vi "FGGA Serial Data Server & Recordingv3.1_test.vi"() -> ()   [LabVIEW 2014]
uses:
  <vilib>/Instr/_visa.llb/VISA Set IO Buffer Mask.ctl
  <vilib>/Instr/_visa.llb/VISA Flush IO Buffer Mask.ctl
  <vilib>/Platform/TimedLoop/XDataNode/timing_clust.ctl
  <vilib>/Platform/TimedLoop/XDataNode/nitl_modes.ctl
  <vilib>/Platform/TimedLoop/XDataNode/wakeup.ctl
  C:/Program Files (x86)/National Instruments/LabVIEW 2014/examples/Data Communication/Network Streams/Simple Network Streams/support/Network Stream Command.ctl
  <vilib>/Utility/error.llb/whitespace.ctl
  <vilib>/Instr/_visa.llb/VISA Configure Serial Port (Instr).vi
  <vilib>/Utility/tcp.llb/UDP Multicast Write-Only Open.vi
  <vilib>/platform/TimedLoop/XDataNode/XDataNode.xnode
  <vilib>/Platform/TimedLoop/XDataNode/XDNodeRunTimeDep.lvlib
panel:
  out "date/time string":string
  out "FGGA Pump":bool
  out "Flight Number":string
  out "Stop File Write":bool
  out "Default file name":string
  out "MFC":dbl[](array[numeric])
  out "FGGA restart":bool
  out "V4":bool
  out "V3":bool
  out "V2":bool
  out "V1":bool
  out "error out 2":errorcluster
  out "error out":errorcluster
  in  "MFC_1 SLPM set value":dbl
  out "Value Read":string
  out "status":bool
  in  "VISA resource name":refnum<visa-resource-name>="ASRL3::INSTR"
  in  "timeout (10sec) 2":u32=3000
  out "Labview_Viewer_UDP_Error_Out":errorcluster
  in  "Clear Display\nErrors":bool
  out "Data Processing":bool
  out "TCP Binary Packet":string
  in  "Time Stamp\nOffset":u32=1
  out "Data String":string
  out "UDP_ACSII_Out":string
  out "Serial error out":errorcluster
  out "SEPTIC TCP Error Out":errorcluster
  out "TCP packet\nSend To SEPTIC":bool
  out "FISH TCP Error Out":errorcluster
  out "TCP packet\nSend To FISH":bool
  out "UDP_Pack_num":u32
  out "UDP_Out Status":bool
  out "UDP_Out_Error Out":errorcluster
  out "Data Array":string[](array[string])
  out "RAW DATA":string
  in  "stop":bool
  in  "timeout (10sec)":u32=1500
  in  "VISA resource name":refnum<visa-resource-name>="ASRL7::INSTR"
  out "Number of times \nRead time out":u32
  out "Loop count":i32
  # "Date"
  # "Time"
  # "CH4"
  # "CO2"
  # "H2O"
  # "Cell Pressure"
  # "Cell Temperature"
  # "Spectral Flag"
  # "Ring Down Time (Laser A)"
  # "Ring Down Time (Laser B)"
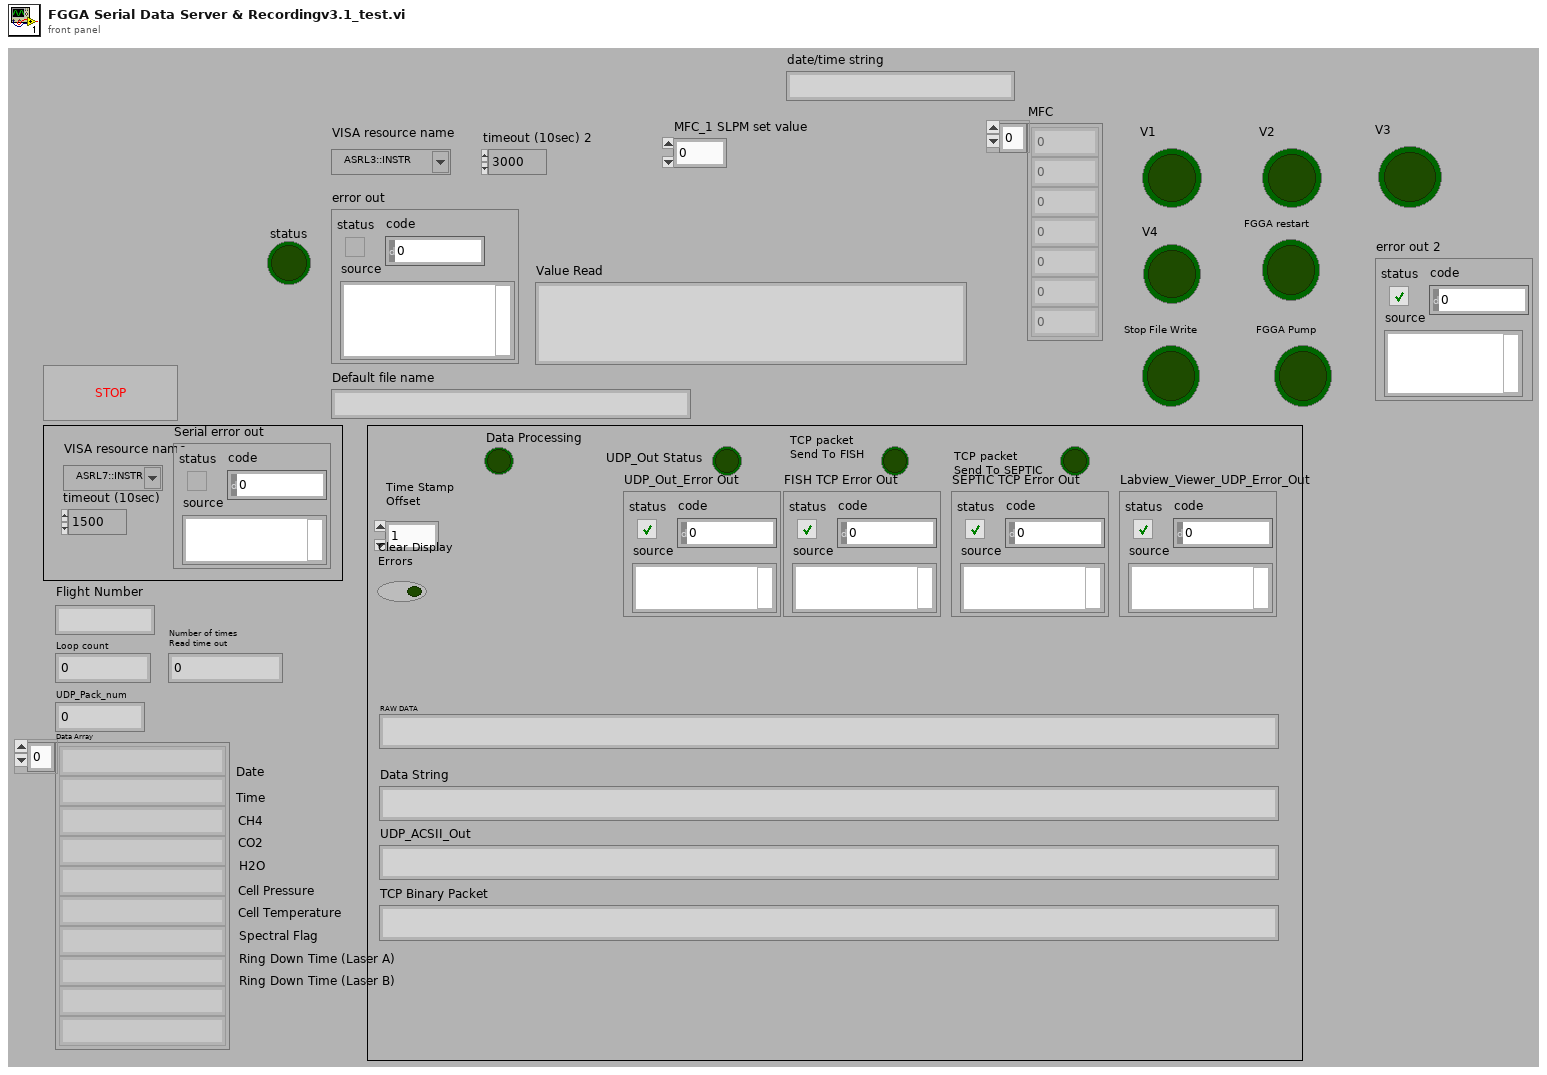
[diagram p1: front panel]
types:
  T1 = typedef "VISA Flush IO Buffer Mask.ctl" = u16
  T2 = typedef "VISA Set IO Buffer Mask.ctl" = u16
  T3 = typedef "XDNodeRunTimeDep.lvlib/timing_clust.ctl" = cluster{"Expected End [f-1]":u64, "Actual End [f-1]":u64, "Finished Late? [f-1]":bool, "Expected End [i-1]":u64, "Actual End [i-1]":u64, "Finished Late? [i-1]":bool, "Expected Start [i]":u64, "Actual Start [i]":u64, "Expected Start [f]":u64, "Actual Start [f]":u64, "Source Name":string, "Structure Name":string, "Period":i64, "Deadline":i64, "Offset":i64, "Start":i64, "Priority":i32, "Timeout":i32, "Mode":T4, "Wakeup Reason":T5, "Error":errorcluster, "Source Type":string, "Secondary Source Type":string, "Global End Time":u64, "Global Start Time":u64, "Frame Duration":u64, "Iteration Duration":u64, "Assigned CPU":i32, "I/O Scan Engine Mode":u32}
  T4 = typedef "XDNodeRunTimeDep.lvlib/nitl_modes.ctl" = enum32{"No Change", "Process missed periods, maintain original phase", "Discard missed periods, maintain original phase", "Process missed periods, ignore original phase", "Discard missed periods, ignore original phase"}
  T5 = typedef "XDNodeRunTimeDep.lvlib/wakeup.ctl" = enum32{"Normal", "Aborted", "Asynchronous wakeup", "Timing source error", "Timed loop error", "Timeout"}
  T6 = typedef "Network Stream Command.ctl" = cluster{"Message":string, "Message Data":variant}
  T7 = enum16{"open", "replace", "create", "open or create", "replace or create", "replace or create with confirmation"}
  T8 = typedef "whitespace.ctl" = u16
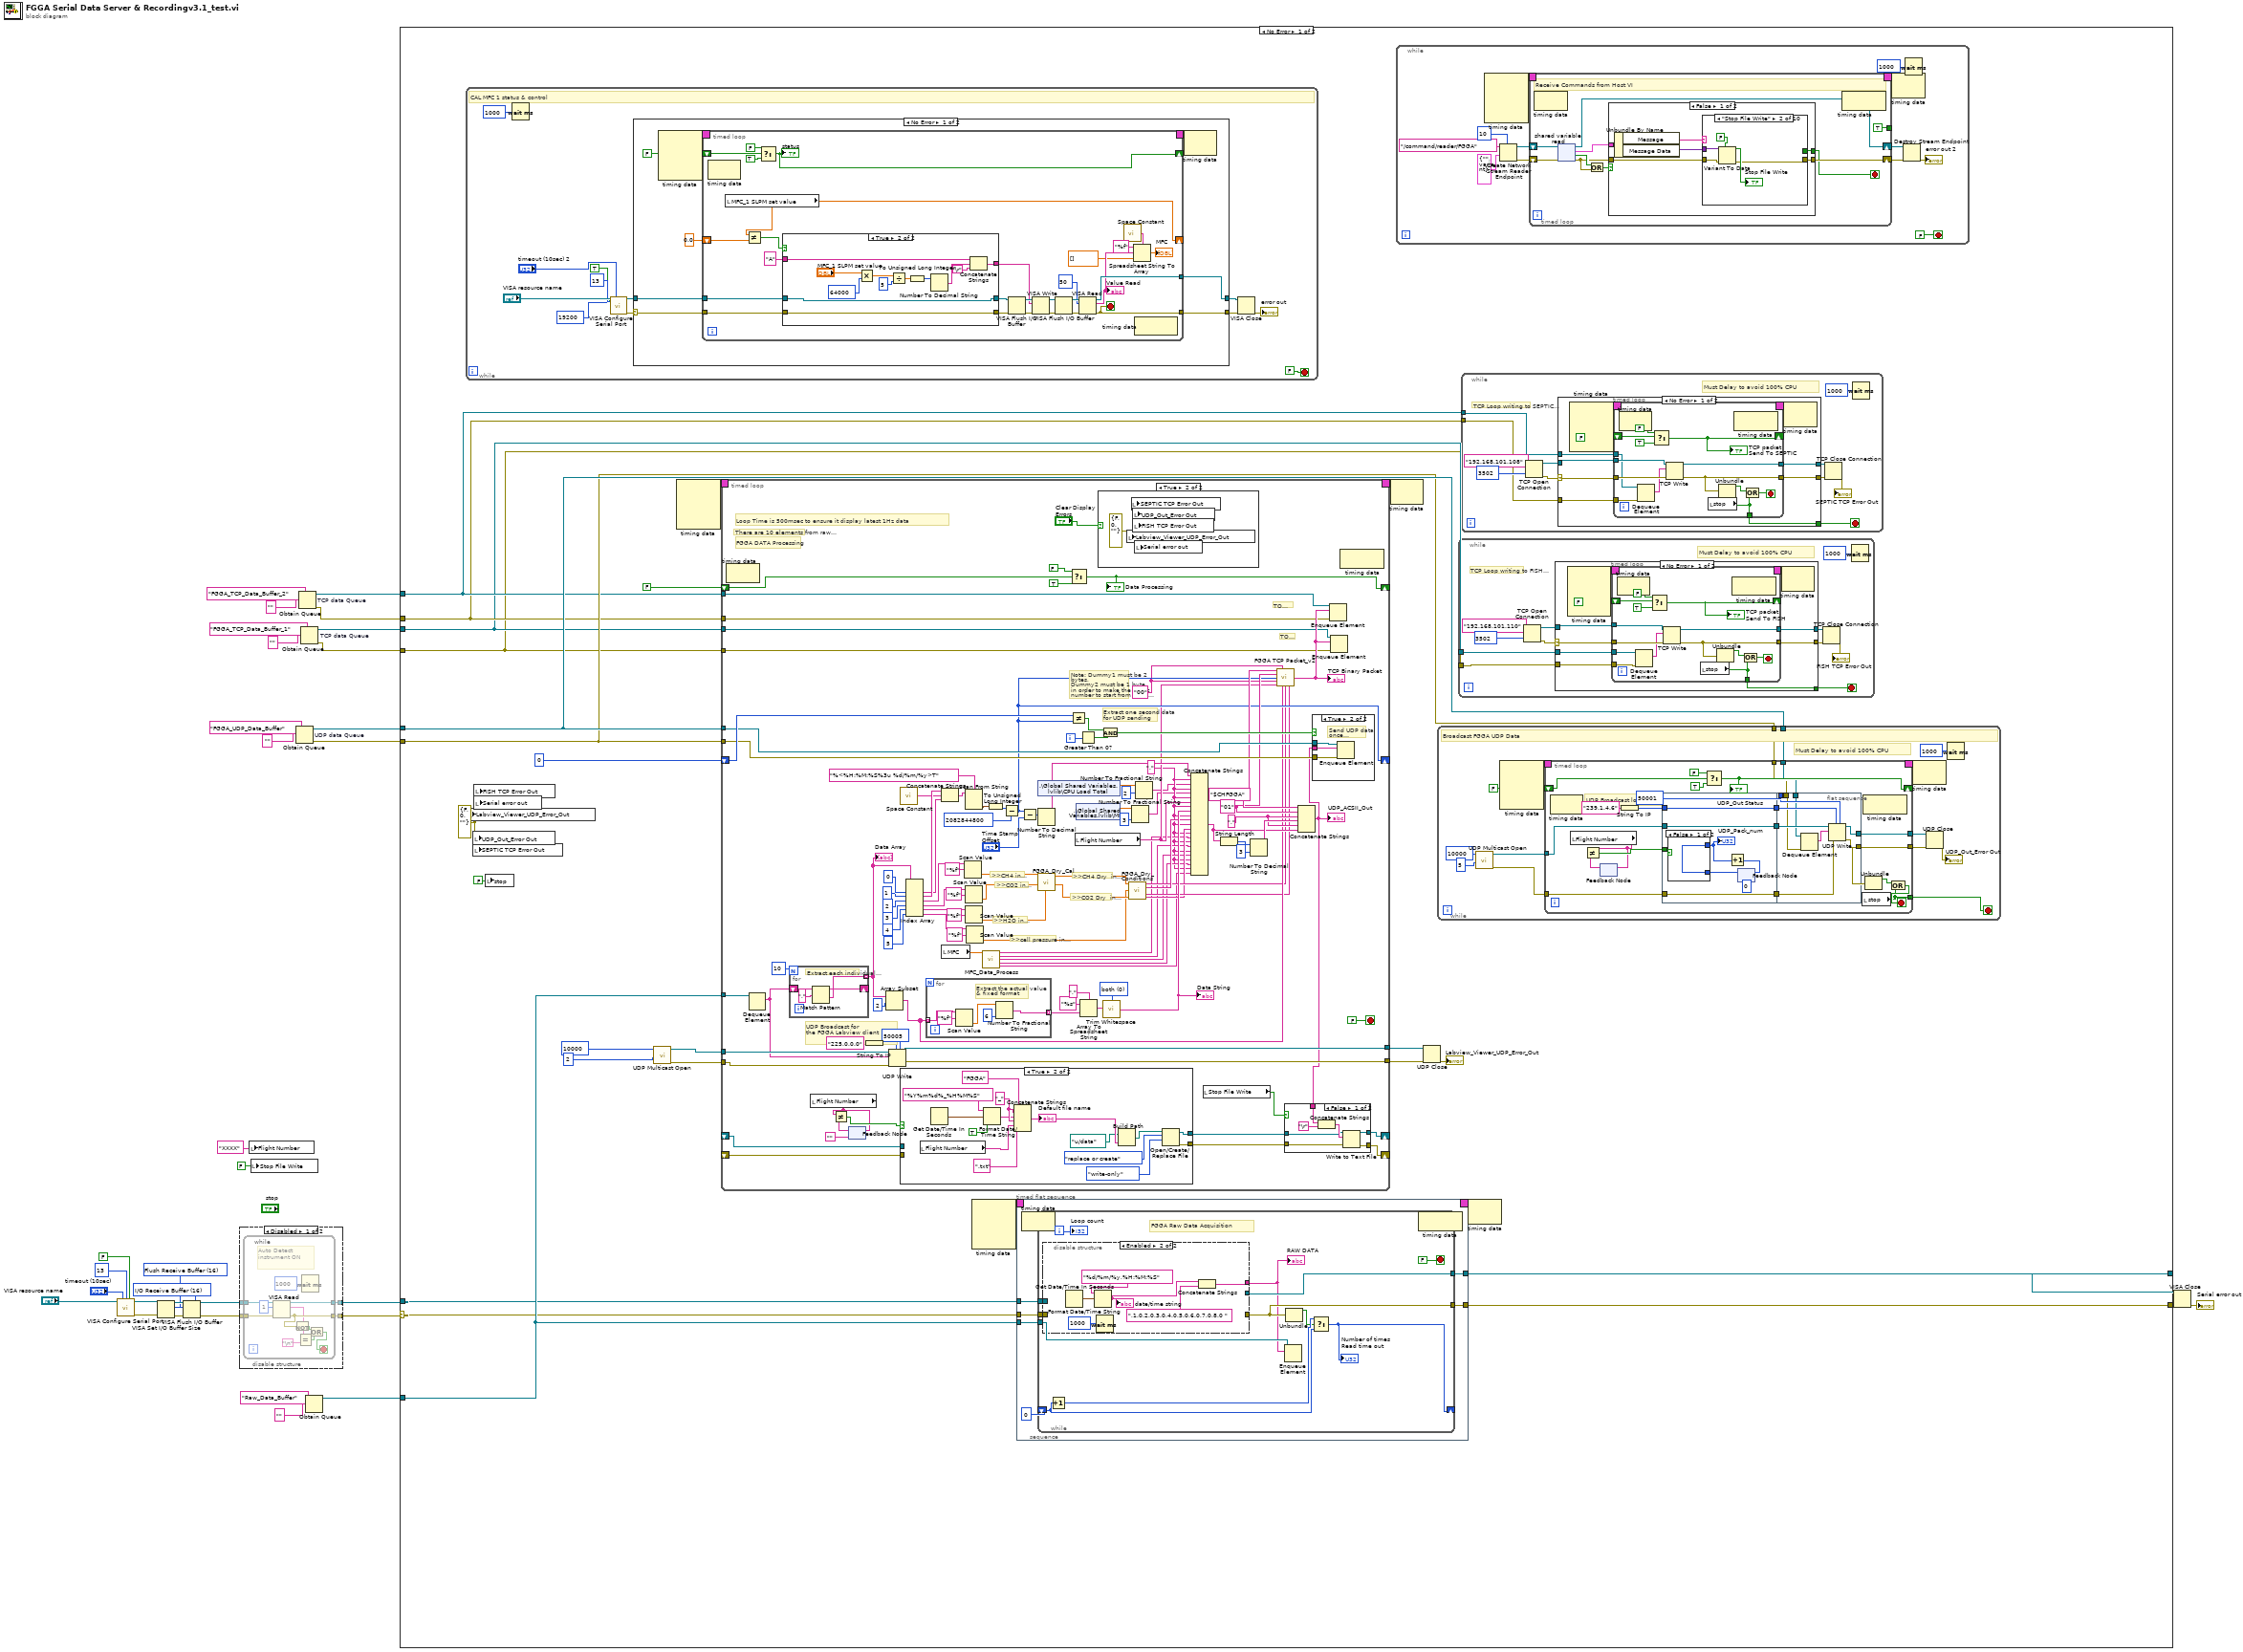
[diagram p0: block diagram]
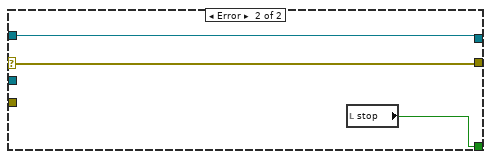
[diagram p3: hidden frame]
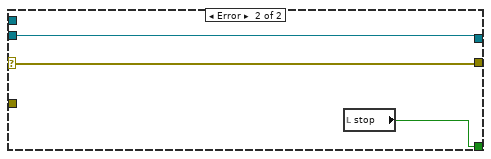
[diagram p4: hidden frame]
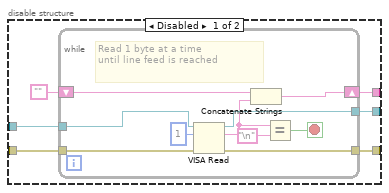
[diagram p5: hidden frame]
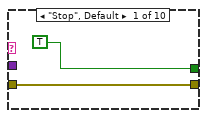
[diagram p6: hidden frame]
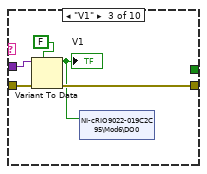
[diagram p7: hidden frame]
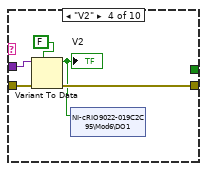
[diagram p8: hidden frame]
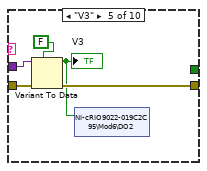
[diagram p9: hidden frame]
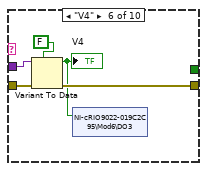
[diagram p10: hidden frame]
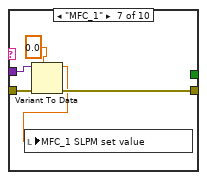
[diagram p11: hidden frame]
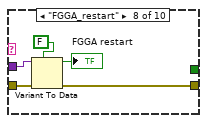
[diagram p12: hidden frame]
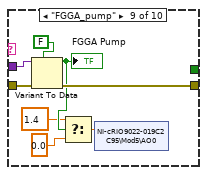
[diagram p13: hidden frame]
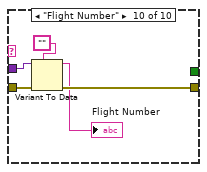
[diagram p14: hidden frame]
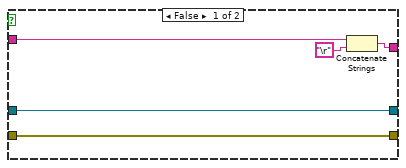
[diagram p16: hidden frame]
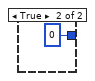
[diagram p18: hidden frame]
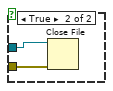
[diagram p20: hidden frame]
diagram:
  w9 = T1 16 items=["Flush Receive Buffer"=16, "Write Transmit Buffer to Device"=32, "Flush Receive Buffer (No I/O)"=64, "Flush Transmit Buffer"=128] ("Mask")
  w10 = T2 16 items=["I/O Receive Buffer"=16, "I/O Transmit Buffer"=32, "I/O Receive and Transmit Buffer"=48] ("Mask")
  n1 = call-poly "VISA Configure Serial Port"("VISA resource name"="VISA resource name", "timeout (10sec)"="timeout (10sec)", "termination char\n(0xA = '\\n' = LF)"=u8 13 ("termination char\n(0xA = '\\n' = LF)"), "Enable Termination\nChar (T)"=FALSE ("Enable Termination\nChar (T)")) -> ("VISA resource name out"=w8:refnum<visa-resource-name>, "error out"=w7:errorcluster)  [unwired: 10 in]
  n2 = VISA Set I/O Buffer Size(VISA resource name=w8, mask (16)=w10, error in (no error)=w7) -> (VISA resource name out=w11:refnum<visa-resource-name>, error out=w12:errorcluster)  [unwired: 1 in]
  n3 = VISA Flush I/O Buffer(VISA resource name=w11, mask (16)=w9, error in (no error)=w12) -> (VISA resource name out=w6:refnum<visa-resource-name>, error out=w5:errorcluster)
  n4 = disable-structure shown="Disabled" {
    disable-tunnel: w6 -> [w38 _]
    disable-tunnel: w5 -> [w37 _]
    disable-tunnel: [w36 _] -> w4
    disable-tunnel: [w35 _] -> w3
    frame Disabled {
      n5 = while {
        tunnel: w38 -> [w49]
        tunnel: w37 -> [w48]
        tunnel: [w46] -> w36
        tunnel: [w45] -> w35
        stop <- w40 stop-if-true
        # "Auto Detect\ninstrument ON"
        n6 = VISA Read(VISA resource name=w49, byte count=u32 1, error in (no error)=w48) -> (VISA resource name out=w45:refnum<visa-resource-name>, read buffer=w43:string, error out=w46:errorcluster)  [unwired: 1 out]
        n7 = Not(x=w46) -> (.not. x?=w42:bool)
        n8 = Equal?(x=w43, y="\n") -> (x = y?=w41:bool)
        n9 = Wait (ms)(milliseconds to wait=u32 1000) -> ()  [unwired: 1 out]
        n10 = Or(x=w42, y=w41) -> (x .or. y?=w40:bool)
      }
    }
    frame Enabled {
    }
  }
  n11 = local write "Flight Number"("XXXX" ("Flight Number")) -> ()
  n12 = local write "Stop File Write"(FALSE ("Stop File Write")) -> ()
  n13 = Obtain Queue "UDP data Queue"(name (unnamed)="FGGA_UDP_Data_Buffer", element data type="") -> (queue out=w22:refnum<queue>, error out=w21:errorcluster)  [unwired: 3 in, 1 out]
  n14 = Obtain Queue "TCP data Queue"(name (unnamed)="FGGA_TCP_Data_Buffer_2", element data type="") -> (queue out=w16:refnum<queue>, error out=w15:errorcluster)  [unwired: 3 in, 1 out]
  n15 = Obtain Queue "TCP data Queue"(name (unnamed)="FGGA_TCP_Data_Buffer_1", element data type="") -> (queue out=w14:refnum<queue>, error out=w13:errorcluster)  [unwired: 3 in, 1 out]
  n16 = Obtain Queue(name (unnamed)="Raw_Data_Buffer", element data type="") -> (queue out=w28:refnum<queue>)  [unwired: 3 in, 2 out]
  n17 = case shown="No Error" w4 {
    selector: w4 -> [w52 w572]
    tunnel: w3 -> [w53 w573]
    tunnel: [w74 w573] -> w25
    tunnel: [w75 w572] -> w26
    tunnel: w28 -> [w71 _]
    tunnel: w22 -> [w69 _]
    tunnel: w21 -> [w68 _]
    tunnel: w16 -> [w67 _]
    tunnel: w15 -> [w66 _]
    tunnel: w14 -> [w65 _]
    tunnel: w13 -> [w64 _]
    frame No Error {
      w55 = errorcluster {"status"=FALSE, "code"=0, "source"=""} ("UDP Error Out")
      n18 = while {
        stop <- FALSE stop-if-true
        # "CAL MFC 1 status & control"
        n19 = Wait (ms)(milliseconds to wait=u32 1000) -> ()  [unwired: 1 out]
        n20 = call-poly "VISA Configure Serial Port"("VISA resource name"="VISA resource name", "timeout (10sec)"="timeout (10sec) 2", "termination char\n(0xA = '\\n' = LF)"=u8 13 ("termination char\n(0xA = '\\n' = LF)"), "Enable Termination\nChar (T)"=TRUE ("Enable Termination\nChar (T)"), "baud rate (9600)"=u32 19200) -> ("VISA resource name out"=w304:refnum<visa-resource-name>, "error out"=w300:errorcluster)  [unwired: 9 in]
        n21 = case shown="No Error" w300 {
          selector: w300 -> [w311 w361]
          tunnel: w304 -> [w312 w362]
          tunnel: [w310 w362] -> w303
          tunnel: [w309 w361] -> w302
          frame No Error {
            n22 = node-c288() -> (w307:T3)  [unwired: 4 in]
            n23 = timed-loop {
              tunnel: w312 -> [w335]
              tunnel: w311 -> [w333]
              tunnel: [w326] -> w310
              tunnel: [w321] -> w309
              shift-right: [w322] -> _
              shift-left: FALSE -> [w325]
              timing: w307 -> [_]
              timing-out: [_] -> w306
              shift-right: [w313] -> _
              shift-left: 0.0 -> [w315]
              stop <- w321 stop-if-true
              n24 = node-c288() -> ()  [unwired: 1 in, 1 out]
              n25 = local read "MFC_1 SLPM set value"() -> (w313:dbl)
              n26 = Not Equal?(x=w313, y=w315) -> (x != y?=w314:bool)
              n27 = Select(t=FALSE, s=w325, f=TRUE) -> (s? t:f=w322:bool)
              "status" <- w322
              n28 = case shown="True" w314 {
                tunnel: w335 -> [w343 w358]
                tunnel: [w343 w358] -> w334
                tunnel: w333 -> [w342 w357]
                tunnel: [w342 w357] -> w332
                tunnel: "A" -> [w346 w350]
                tunnel: [w344 w347] -> w330
                frame False {
                  n29 = Concatenate Strings(w346, "\r") -> (w344:string)
                }
                frame True {
                  n30 = Multiply(x="MFC_1 SLPM set value", y=u32 64000) -> (x*y=w354:dbl)
                  n31 = Divide(x=w354, y=u32 5) -> (x/y=w352:dbl)
                  n32 = To Unsigned Long Integer(number=w352) -> (unsigned 32bit integer=w351:u32)
                  n33 = Number To Decimal String(number=w351) -> (decimal integer string=w349:string)  [unwired: 1 in]
                  n34 = Concatenate Strings(w350, w349, "\r") -> (w347:string)
                }
              }
              n35 = VISA Flush I/O Buffer(VISA resource name=w334, error in (no error)=w332) -> (VISA resource name out=w337:refnum<visa-resource-name>, error out=w336:errorcluster)  [unwired: 1 in]
              n36 = VISA Write(VISA resource name=w337, write buffer=w330, error in (no error)=w336) -> (VISA resource name out=w329:refnum<visa-resource-name>, error out=w328:errorcluster)  [unwired: 1 out]
              n37 = VISA Flush I/O Buffer(VISA resource name=w329, error in (no error)=w328) -> (VISA resource name out=w339:refnum<visa-resource-name>, error out=w338:errorcluster)  [unwired: 1 in]
              n38 = VISA Read(VISA resource name=w339, byte count=u32 50, error in (no error)=w338) -> (VISA resource name out=w326:refnum<visa-resource-name>, read buffer=w320:string, error out=w321:errorcluster)  [unwired: 1 out]
              "Value Read" <- w320
              n39 = call <vilib>:"Space Constant.vi"() -> ("String"=w319:string)
              n40 = Spreadsheet String To Array(delimiter (Tab)=w319, format string="%f", spreadsheet string=w320, array type (2D Dbl)=dbl[] []) -> (array=→"MFC":dbl[])
              n41 = node-c288() -> ()  [unwired: 1 in, 1 out]
            }
            n42 = node-c288(w306) -> ()  [unwired: 1 out]
          }
          frame Error {
          }
        }
        n43 = VISA Close(VISA resource name=w303, error in (no error)=w302) -> (error out=→"error out":errorcluster)
      }
      n44 = local write "Labview_Viewer_UDP_Error_Out"(w55) -> ()
      n45 = local write "UDP_Out_Error Out"(w55) -> ()
      n46 = local write "SEPTIC TCP Error Out"(w55) -> ()
      n47 = local write "FISH TCP Error Out"(w55) -> ()
      n48 = local write "Serial error out"(w55) -> ()
      n49 = local write "stop"(FALSE ("stop")) -> ()
      n50 = call-poly <vilib>:"UDP Multicast Open.vi"("time-to-live (1)"=u16 2, "port"=u16 10000) -> ("error out"=w59:errorcluster, "connection ID"=w60:refnum<k16>)  [unwired: 8 in]
      n51 = node-c288() -> (w73:T3)  [unwired: 4 in]
      n52 = timed-loop {
        timing: w73 -> [_]
        timing-out: [_] -> w72
        tunnel: w71 -> [w528]
        tunnel: w69 -> [w483]
        tunnel: w68 -> [w482]
        shift-right: [w479] -> _
        shift-left: u32 0 -> [w486]
        tunnel: w67 -> [w474]
        tunnel: w66 -> [w473]
        tunnel: w65 -> [w472]
        tunnel: w64 -> [w471]
        shift-right: [w467] -> _
        shift-left: FALSE -> [w470]
        tunnel: w60 -> [w463]
        tunnel: w59 -> [w462]
        tunnel: [w461] -> w58
        tunnel: [w460] -> w57
        shift-right: [w439] -> _
        shift-left: _ -> [w431]
        shift-right: [w429] -> _
        shift-left: _ -> [w430]
        i -> [w485]
        stop <- FALSE stop-if-true
        w478 = "00"
        w441 = ","
        w514 = T8 0 items=["both", "start of string", "end of string"] ("location (both)")
        w522 = ","
        w480 = "01"
        w481 = "$CHFGGA"
        # "Note: Dummy1 must be 2 bytes, \nDummy2 must be 1 byte\nin order to make the Flight \nnumber to start from byte 20\n(this only applies to TCP packet)"
        # ">>cell pressure in torr>>"
        # "UDP Broadcast for\nthe FGGA Labview client"
        # "There are 10 elements from raw packet"
        # "TO SEPTIC"
        # "TO FISH"
        # "Extract one second data\nfor UDP sending"
        # ">>CO2 Dry  in ppm>>"
        # ">>CH4 Dry  in ppb>>"
        # ">>H2O in ppm>>"
        # ">>CO2 in ppm>>"
        # ">>CH4 in ppm>>"
        # "Loop Time is 500msec to ensure it display latest 1Hz data"
        # "FGGA DATA Processing"
        n53 = node-c288() -> ()  [unwired: 1 in, 1 out]
        n54 = Dequeue Element(queue=w528) -> (element=w459:string)  [unwired: 2 in, 3 out]
        n55 = for {
          N: 10 -> [_]
          shift-right: [w566] -> _
          shift-left: w459 -> [w564]
          tunnel: [w565] -> w519 mode=indexing
          # "Extract each individual param"
          n56 = Match Pattern(string=w564, regular expression=",") -> (before substring=w565:string, after substring=w566:string)  [unwired: 1 in, 2 out]
        }
        "Data Array" <- w519
        n57 = local read "Flight Number"() -> (w428:string)
        n58 = feedback #1("" ("Flight Number")) -> (w436:string)
        n59 = Not Equal?(x=w428, y=w436) -> (x != y?=w434:bool)
        n60 = feedback-in #1(w428) -> ()
        n61 = String To IP(1:"225.0.0.0" ("name")) -> (0:w464:u32)
        n62 = Array Subset(array=w519, index=2) -> (w476:string[])  [unwired: 1 in]
        n63 = UDP Write(address=w464, port or service name=u16 50005, connection ID=w463, data in=w459, 8:w462) -> (error out=w460:errorcluster, 3:w461:refnum<k16>)  [unwired: 1 in]
        n64 = case shown="True" w434 {
          tunnel: [w530 w532] -> w433
          tunnel: [w529 w531] -> w432
          tunnel: w431 -> [w530 _]
          tunnel: w430 -> [w529 _]
          frame False {
          }
          frame True {
            w538 = "_" ("string")
            n65 = local read "Flight Number"() -> (w545:string)
            n66 = Get Date/Time In Seconds() -> (seconds since 1Jan1904=w533:timestamp)
            n67 = Format Date/Time String(time format string (%c)="%Y%m%d%_%H%M%S", seconds (now)=w533, UTC format=TRUE) -> (date/time string=w535:string)
            n68 = Concatenate Strings("FGGA" ("string"), w538, w535, w538, w545, ".txt" ("string")) -> (w540:string)
            "Default file name" <- w540
            n69 = Build Path(base path=path "u:/data", name or relative path=w540) -> (appended path=w544:path)
            n70 = Open/Create/Replace File(file path (use dialog)=w544, operation (0:open)=T7."replace or create", access (0:read/write)=enum16{"read/write", "read-only", "write-only"}."write-only") -> (refnum out=w532:refnum<file>, error out=w531:errorcluster)  [unwired: 3 in, 1 out]
          }
        }
        n71 = call <vilib>:"Space Constant.vi"() -> ("String"=w497:string)
        n72 = Index Array(array=w519, index #1=0 ("index"), index #2=1 ("index"), index #3=2 ("index"), index #4=3 ("index"), index #5=4 ("index"), index #6=5 ("index")) -> (element #1=w496:string, element #2=w498:string, element #3=w502:string, element #4=w501:string, element #5=w500:string, element #6=w450:string)
        n73 = for {
          tunnel: w476 -> [w562] mode=indexing
          tunnel: [w559] -> w512 mode=indexing
          # "Extract the actual value\n& fixed format"
          n74 = Scan Value(string=w562, format string="%f") -> (value=w560:dbl)  [unwired: 1 in, 1 out]
          n75 = Number To Fractional String(number=w560, precision (6)=i16 6) -> (F-format string=w559:string)  [unwired: 2 in]
        }
        n76 = Concatenate Strings(w498, w497, w496) -> (w495:string)
        n77 = local read "MFC"() -> (w446:dbl[])
        n78 = Scan Value(string=w502, format string="%f") -> (value=w504:dbl)  [unwired: 1 in, 1 out]
        n79 = Scan Value(string=w501, format string="%f") -> (value=w503:dbl)  [unwired: 1 in, 1 out]
        n80 = Scan From String(format string="%<%H:%M:%S%3u %d/%m/%y>T", input string=w495) -> (output 1=w492:timestamp)  [unwired: 3 in, 3 out]
        n81 = Scan Value(string=w500, format string="%f") -> (value=w447:dbl)  [unwired: 1 in, 1 out]
        n82 = Scan Value(string=w450, format string="%f") -> (value=w448:dbl)  [unwired: 1 in, 1 out]
        n83 = call "MFC_Data_Process.vi"("MFC"=w446) -> ("MFC Absolute Pressure"=w445:string, "MFC Temperature"=w444:string, "MFC Volumetric Flow"=w443:string, "MFC Mass Flow"=w442:string, "MFC Set Point"=w440:string)  [unwired: 10 in]
        n84 = To Unsigned Long Integer(number=w492) -> (unsigned 32bit integer=w493:u32)
        n85 = Subtract(x=w493, y=u32 2082844800) -> (x-y=w479:u32)
        n86 = Subtract(x=w479, y="Time Stamp\nOffset") -> (x-y=w489:u32)
        n87 = shared-variable ".\\Global Shared Variables.lvlib\\CPU Load Total"() -> (w427:dbl)  [unwired: 1 in, 1 out]
        n88 = Number To Decimal String(number=w489) -> (decimal integer string=w491:string)  [unwired: 1 in]
        n89 = call "FGGA_Dry_Cal.vi"("H2O"=w447, "CO2_Wet"=w503, "CH4_Wet"=w504) -> ("CO2_Dry"=w452:dbl, "CH4_Dry"=w454:dbl)  [unwired: 7 in]
        n90 = Select(t=FALSE, s=w470, f=TRUE) -> (s? t:f=w467:bool)
        "Data Processing" <- w467
        n91 = Not Equal?(x=w486, y=w479) -> (x != y?=w487:bool)
        n92 = local read "Flight Number"() -> (w477:string)
        n93 = shared-variable ".\\Global Shared Variables.lvlib\\MFM"() -> (w424:dbl)  [unwired: 1 in, 1 out]
        n94 = Greater Than 0?(x=w485) -> (x > 0?=w488:bool)
        n95 = Array To Spreadsheet String(delimiter (Tab)=",", array=w512, 3:"%s" ("format string")) -> (spreadsheet string=w513:string)
        n96 = case shown="True" "Clear Display\nErrors" {
          frame False {
          }
          frame True {
            w555 = errorcluster {"status"=FALSE, "code"=0, "source"=""} ("UDP Error Out")
            n97 = local write "Labview_Viewer_UDP_Error_Out"(w555) -> ()
            n98 = local write "SEPTIC TCP Error Out"(w555) -> ()
            n99 = local write "UDP_Out_Error Out"(w555) -> ()
            n100 = local write "FISH TCP Error Out"(w555) -> ()
            n101 = local write "Serial error out"(w555) -> ()
          }
        }
        n102 = call <vilib>:"Trim Whitespace.vi"("string"=w513, "location (both)"=w514) -> ("trimmed string"=w511:string)
        "Data String" <- w511
        n103 = Compound Arithmetic op=AND(w487, w488) -> (w484:bool)
        n104 = call "FGGA_Dry_Conditions.vi"("CH4_Dry"=w454, "Pressure"=w448, "CO2_Dry"=w452) -> ("CH4_Dry_TCP"=w457:string, "CH4_Dry_UDP"=w458:string, "CO2_Dry_TCP"=w456:string, "CO2_Dry_UDP"=w455:string)  [unwired: 9 in]
        n105 = Number To Fractional String(number=w424, precision (6)=i16 3) -> (F-format string=w422:string)  [unwired: 2 in]
        n106 = Number To Fractional String(number=w427, precision (6)=i16 2) -> (F-format string=w425:string)  [unwired: 2 in]
        n107 = Concatenate Strings(w491, w441, w425, w441, w422, w441, w477, w441, w511, w441, w458, w441, w455, w441, w445, w441, w444, w441, w443, w441, w442, w441, w440) -> (w521:string)
        n108 = local read "Stop File Write"() -> (w437:bool)
        n109 = String Length(string=w521) -> (length=w525:i32)
        n110 = Number To Decimal String(number=w525, width (-)=i16 3) -> (decimal integer string=w523:string)
        n111 = call "FGGA TCP Packet_v2.vi"("ID"=w481, "dummy2"=w478, "Version"=w480, "utc_time"=w479, "dummy1"=w478, "Flight Number"=w477, "Data Array"=w476, "ch4_dry"=w457, "co2_dry"=w456) -> ("TCP Binary Packet"=w475:string)  [unwired: 6 in]
        "TCP Binary Packet" <- w475
        n112 = Concatenate Strings(w481, w480, w522, w523, w522, w521) -> (w438:string)
        "UDP_ACSII_Out" <- w438
        n113 = case shown="False" w437 {
          tunnel: w438 -> [w552 _]
          tunnel: [w549 _] -> w439
          tunnel: w433 -> [w548 w554]
          tunnel: w432 -> [w547 w553]
          tunnel: [w546 _] -> w429
          frame False {
            n114 = Concatenate Strings(w552, "\r") -> (w550:string)
            n115 = Write to Text File(file (use dialog)=w548, text=w550, error in=w547) -> (refnum out=w549:refnum<file>, error out=w546:errorcluster)  [unwired: 2 out]
          }
          frame True {
            n116 = Close File(refnum=w554, error in=w553) -> ()  [unwired: 2 out]
          }
        }
        n117 = case shown="True" w484 {
          tunnel: w438 -> [_ w558]
          tunnel: w483 -> [_ w557]
          tunnel: w482 -> [_ w556]
          frame False {
          }
          frame True {
            # "Send UDP data once\na second"
            n118 = Enqueue Element(queue=w557, element=w558, error in (no error)=w556) -> ()  [unwired: 1 in, 3 out]
          }
        }
        n119 = Enqueue Element(queue=w474, element=w475, error in (no error)=w473) -> ()  [unwired: 1 in, 3 out]
        n120 = Enqueue Element(queue=w472, element=w475, error in (no error)=w471) -> ()  [unwired: 1 in, 3 out]
        n121 = node-c288() -> ()  [unwired: 1 in, 1 out]
      }
      n122 = node-c288() -> (w51:T3)  [unwired: 4 in]
      n123 = timed-sequence {
        timing: w51 -> [_]
        timing-out: [_] -> w50
        tunnel: [w164] -> w75
        tunnel: [w163] -> w74
        tunnel: w71 -> [w162]
        tunnel: w53 -> [w161]
        tunnel: w52 -> [w160]
        n124 = timed-flat-sequence {
          tunnel: [w170] -> w164
          tunnel: [w169] -> w163
          tunnel: w162 -> [w167]
          tunnel: w161 -> [w166]
          tunnel: w160 -> [w165]
          n125 = node-c288() -> ()  [unwired: 1 in, 1 out]
          n126 = while {
            tunnel: w166 -> [w182]
            tunnel: w165 -> [w181]
            tunnel: [w180] -> w170
            shift-right: [w176] -> _
            shift-left: u32 0 -> [w177]
            tunnel: [w179] -> w169
            tunnel: w167 -> [w174]
            i -> [w178]
            stop <- FALSE stop-if-true
            # "FGGA Raw Data Acquisition"
            n127 = disable-structure shown="Enabled" {
              disable-tunnel: w182 -> [w188 _]
              disable-tunnel: w181 -> [w187 _]
              disable-tunnel: [w186 _] -> w180
              disable-tunnel: [w185 _] -> w179
              disable-tunnel: [w183 w200] -> w173
              frame Disabled {
                n128 = while {
                  tunnel: [w198] -> w185
                  tunnel: [w197] -> w186
                  tunnel: w188 -> [w196]
                  tunnel: w187 -> [w195]
                  shift-right: [w193] -> w183
                  shift-left: "" -> [w194]
                  stop <- w190 stop-if-true
                  # "Read 1 byte at a time \nuntil line feed is reached"
                  n129 = VISA Read(VISA resource name=w196, byte count=u32 1, error in (no error)=w195) -> (VISA resource name out=w198:refnum<visa-resource-name>, read buffer=w192:string, error out=w197:errorcluster)  [unwired: 1 out]
                  n130 = Concatenate Strings(w194, w192) -> (w193:string)
                  n131 = Equal?(x=w192, y="\n") -> (x = y?=w190:bool)
                }
              }
              frame Enabled {
                n132 = Get Date/Time In Seconds() -> (seconds since 1Jan1904=w203:timestamp)
                n133 = Format Date/Time String(time format string (%c)="%d/%m/%y,%H:%M:%S" ("format string"), seconds (now)=w203) -> (date/time string=w199:string)  [unwired: 1 in]
                "date/time string" <- w199
                n134 = Wait (ms)(milliseconds to wait=u32 1000) -> ()  [unwired: 1 out]
                n135 = Concatenate Strings(w199, ",1.0,2.0,3.0,4.0,5.0,6.0,7.0,8.0 " ("RAW DATA")) -> (w200:string)
              }
            }
            "RAW DATA" <- w173
            n136 = Increment(x=w177) -> (x+1=w175:u32)
            n137 = Enqueue Element(queue=w174, element=w173) -> ()  [unwired: 2 in, 3 out]
            n138 = Unbundle(w180) -> ("status"=w172:bool)  [unwired: 2 out]
            n139 = Select(t=w175, s=w172, f=w177) -> (s? t:f=w176:u32)
            "Number of times \nRead time out" <- w176
            "Loop count" <- w178
          }
          n140 = node-c288() -> ()  [unwired: 1 in, 1 out]
        }
      }
      n141 = node-c288(w72) -> ()  [unwired: 1 out]
      n142 = while {
        stop <- FALSE stop-if-true
        n143 = node-c288() -> (w210:T3)  [unwired: 4 in]
        n144 = Create Network Stream Reader Endpoint(7:10 ("reader buffer size"), 9:T6 {"Message"="", "Message Data"=variant} ("Message Cluster"), 11:"/command/reader/FGGA" ("reader url")) -> (0:w216:errorcluster, 3:w217:refnum<k21>)  [unwired: 4 in]
        n145 = timed-loop "Host->Target Command Reader" {
          shift-right: [w227] -> w214
          shift-left: w216 -> [w230]
          shift-right: [w228] -> w213
          shift-left: w217 -> [w229]
          tunnel: [TRUE] -> _
          timing: w210 -> [_]
          timing-out: [_] -> w209
          stop <- w221 stop-if-true
          # "Receive Commands from Host VI"
          n146 = node-c288() -> ()  [unwired: 1 in, 1 out]
          n147 = shared-variable-read(w229, w230) -> (w228:refnum<k21>, w223:errorcluster, w225:bool, w226:T6)  [unwired: 1 in]
          n148 = Or(x=w225, y=w223) -> (x .or. y?=w224:bool)
          n149 = case shown="False" w224 {
            selector: w224 -> [_ w289]
            tunnel: w223 -> [w238 w290]
            tunnel: [w237 w290] -> w227
            tunnel: w226 -> [w235 _]
            tunnel: [w236 w289] -> w221
            frame False {
              n150 = Unbundle By Name(w235) -> ("Message"=w234:string, "Message Data"=w233:variant)
              n151 = case shown="\"Stop File Write\"" w234 {
                tunnel: w238 -> [w240 w245 w250 w255 w260 w265 w270 w275 w283 w288]
                tunnel: [w240 w241 w249 w254 w259 w264 w269 w274 w282 w287] -> w237
                tunnel: w233 -> [_ w244 w248 w253 w258 w263 w268 w273 w281 w286]
                tunnel: [TRUE _ _ _ _ _ _ _ _ _] -> w236
                frame "Stop", Default {
                }
                frame "Stop File Write" {
                  n152 = Variant To Data(error in=w245, type=FALSE, Variant=w244) -> (data=→"Stop File Write":bool, error out=w241:errorcluster)
                }
                frame "V1" {
                  n153 = Variant To Data(error in=w250, type=FALSE, Variant=w248) -> (data=w246:bool, error out=w249:errorcluster)
                  "V1" <- w246
                  n154 = shared-variable "NI-cRIO9022-019C2C95\\Mod6\\DO0"(w246) -> ()  [unwired: 1 in, 1 out]
                }
                frame "V2" {
                  n155 = Variant To Data(error in=w255, type=FALSE, Variant=w253) -> (data=w251:bool, error out=w254:errorcluster)
                  "V2" <- w251
                  n156 = shared-variable "NI-cRIO9022-019C2C95\\Mod6\\DO1"(w251) -> ()  [unwired: 1 in, 1 out]
                }
                frame "V3" {
                  n157 = Variant To Data(error in=w260, type=FALSE, Variant=w258) -> (data=w256:bool, error out=w259:errorcluster)
                  "V3" <- w256
                  n158 = shared-variable "NI-cRIO9022-019C2C95\\Mod6\\DO2"(w256) -> ()  [unwired: 1 in, 1 out]
                }
                frame "V4" {
                  n159 = Variant To Data(error in=w265, type=FALSE, Variant=w263) -> (data=w261:bool, error out=w264:errorcluster)
                  "V4" <- w261
                  n160 = shared-variable "NI-cRIO9022-019C2C95\\Mod6\\DO3"(w261) -> ()  [unwired: 1 in, 1 out]
                }
                frame "MFC_1" {
                  n161 = Variant To Data(error in=w270, type=0.0, Variant=w268) -> (data=w266:dbl, error out=w269:errorcluster)
                  n162 = local write "MFC_1 SLPM set value"(w266) -> ()
                }
                frame "FGGA_restart" {
                  n163 = Variant To Data(error in=w275, type=FALSE, Variant=w273) -> (data=→"FGGA restart":bool, error out=w274:errorcluster)
                }
                frame "FGGA_pump" {
                  n164 = Variant To Data(error in=w283, type=FALSE, Variant=w281) -> (data=w278:bool, error out=w282:errorcluster)
                  "FGGA Pump" <- w278
                  n165 = Select(t=1.4 ("f"), s=w278, f=0.0 ("t")) -> (s? t:f=w279:dbl)
                  n166 = shared-variable "NI-cRIO9022-019C2C95\\Mod5\\AO0"(w279) -> ()  [unwired: 1 in, 1 out]
                }
                frame "Flight Number" {
                  n167 = Variant To Data(error in=w288, type="", Variant=w286) -> (data=→"Flight Number":string, error out=w287:errorcluster)
                }
              }
            }
            frame True {
            }
          }
          n168 = node-c288() -> ()  [unwired: 1 in, 1 out]
        }
        n169 = node-c288(w209) -> ()  [unwired: 1 out]
        n170 = Destroy Stream Endpoint(8:w214, 11:w213) -> (0:→"error out 2":errorcluster)
        n171 = Wait (ms)(milliseconds to wait=u32 1000) -> ()  [unwired: 1 out]
      }
      n172 = UDP Close(connection ID=w58, 8:w57) -> (error out=→"Labview_Viewer_UDP_Error_Out":errorcluster)  [unwired: 1 out]
      n173 = while {
        tunnel: w69 -> [w365]
        tunnel: w68 -> [w364]
        stop <- w366 stop-if-true
        # "Must Delay to avoid 100% CPU"
        # "Broadcast FGGA UDP Data"
        n174 = call-poly <vilib>:"UDP Multicast Open.vi"("time-to-live (1)"=u16 5, "port"=u16 10000) -> ("error out"=w373:errorcluster, "connection ID"=w374:refnum<k16>)  [unwired: 8 in]
        n175 = node-c288() -> (w376:T3)  [unwired: 4 in]
        n176 = timed-loop {
          tunnel: w374 -> [w397]
          tunnel: w373 -> [w396]
          timing: w376 -> [_]
          timing-out: [_] -> w375
          shift-right: [w385] -> _
          shift-left: FALSE -> [w388]
          tunnel: [w384] -> w368
          tunnel: [w382] -> w367
          tunnel: [w380] -> w366
          tunnel: w365 -> [w378]
          tunnel: w364 -> [w377]
          stop <- w381 stop-if-true
          # "UDP Broadcast loop"
          n177 = node-c288() -> ()  [unwired: 1 in, 1 out]
          n178 = local read "Flight Number"() -> (w379:string)
          n179 = feedback-in #2(w379) -> ()
          n180 = feedback #2() -> (w390:string)  [unwired: 1 in]
          n181 = Not Equal?(x=w379, y=w390) -> (x != y?=w389:bool)
          n182 = String To IP(1:"239.1.4.6" ("name")) -> (0:w394:u32)
          n183 = flat-sequence {
            tunnel: w394 -> [w404]
            tunnel: w396 -> [w405]
            tunnel: w397 -> [w406]
            tunnel: [w406] -> w393
            tunnel: [w405] -> w392
            tunnel: [w404] -> w391
            tunnel: w389 -> [w403]
            tunnel: u16 50001 ("port or service name") -> [w417]
            tunnel: w393 -> [w416]
            tunnel: w392 -> [w415]
            tunnel: w391 -> [w414]
            tunnel: [w413] -> w384
            tunnel: [w412] -> w382
            tunnel: w378 -> [w410]
            tunnel: w377 -> [w409]
            frame #0 {
              n184 = feedback #3(u32 0) -> (w400:u32)
              n185 = case shown="False" w403 {
                tunnel: w400 -> [w407 _]
                tunnel: [w407 u32 0] -> w399
                frame False {
                }
                frame True {
                }
              }
              "UDP_Pack_num" <- w399
              n186 = Increment(x=w399) -> (x+1=w401:u32)
              n187 = feedback-in #3(w401) -> ()
            }
            frame #1 {
              n188 = Dequeue Element(queue=w410, error in (no error)=w409) -> (element=w411:string)  [unwired: 1 in, 3 out]
              n189 = UDP Write(address=w414, port or service name=w417, connection ID=w416, data in=w411, 8:w415) -> (error out=w412:errorcluster, 3:w413:refnum<k16>)  [unwired: 1 in]
            }
          }
          n190 = Select(t=FALSE, s=w388, f=TRUE) -> (s? t:f=w385:bool)
          "UDP_Out Status" <- w385
          n191 = local read "stop"() -> (w380:bool)
          n192 = node-c288() -> ()  [unwired: 1 in, 1 out]
          n193 = Unbundle(w382) -> ("status"=w383:bool)  [unwired: 2 out]
          n194 = Compound Arithmetic op=OR(w383, w380) -> (w381:bool)
        }
        n195 = node-c288(w375) -> ()  [unwired: 1 out]
        n196 = UDP Close(connection ID=w368, 8:w367) -> (error out=→"UDP_Out_Error Out":errorcluster)  [unwired: 1 out]
        n197 = Wait (ms)(milliseconds to wait=u32 1000) -> ()  [unwired: 1 out]
      }
      n198 = while {
        tunnel: w65 -> [w78]
        tunnel: w64 -> [w77]
        stop <- w81 stop-if-true
        # "Must Delay to avoid 100% CPU"
        # "TCP Loop writing to FISH Tank"
        n199 = TCP Open Connection(address="192.168.101.110", remote port or service name=u16 3502) -> (connection ID=w84:refnum<k5>, error out=w79:errorcluster)  [unwired: 3 in]
        n200 = case shown="No Error" w79 {
          selector: w79 -> [w89 w116]
          tunnel: w84 -> [w94 w117]
          tunnel: [w93 w117] -> w83
          tunnel: [w92 w116] -> w82
          tunnel: [w91 w115] -> w81
          tunnel: w78 -> [w88 _]
          tunnel: w77 -> [w87 _]
          frame No Error {
            n201 = node-c288() -> (w96:T3)  [unwired: 4 in]
            n202 = timed-loop {
              tunnel: w94 -> [w110]
              tunnel: w89 -> [w109]
              tunnel: [w108] -> w93
              tunnel: [w107] -> w92
              tunnel: [w99] -> w91
              shift-right: [w101] -> _
              shift-left: FALSE -> [w104]
              timing: w96 -> [_]
              timing-out: [_] -> w95
              tunnel: w88 -> [w98]
              tunnel: w87 -> [w97]
              stop <- w105 stop-if-true
              n203 = node-c288() -> ()  [unwired: 1 in, 1 out]
              n204 = Dequeue Element(queue=w98, error in (no error)=w97) -> (element=w100:string)  [unwired: 1 in, 3 out]
              n205 = Select(t=FALSE, s=w104, f=TRUE) -> (s? t:f=w101:bool)
              "TCP packet\nSend To FISH" <- w101
              n206 = TCP Write(connection ID=w110, data in=w100, error in (no error)=w109) -> (connection ID out=w108:refnum<k5>, error out=w107:errorcluster)  [unwired: 1 in, 1 out]
              n207 = local read "stop"() -> (w99:bool)
              n208 = Unbundle(w107) -> ("status"=w106:bool)  [unwired: 2 out]
              n209 = node-c288() -> ()  [unwired: 1 in, 1 out]
              n210 = Compound Arithmetic op=OR(w106, w99) -> (w105:bool)
            }
            n211 = node-c288(w95) -> ()  [unwired: 1 out]
          }
          frame Error {
            n212 = local read "stop"() -> (w115:bool)
          }
        }
        n213 = TCP Close Connection(connection ID=w83, error in (no error)=w82) -> (error out=→"FISH TCP Error Out":errorcluster)  [unwired: 1 in, 1 out]
        n214 = Wait (ms)(milliseconds to wait=u32 1000) -> ()  [unwired: 1 out]
      }
      n215 = while {
        tunnel: w67 -> [w120]
        tunnel: w66 -> [w119]
        stop <- w123 stop-if-true
        # "Must Delay to avoid 100% CPU"
        # "TCP Loop writing to SEPTIC Tank"
        n216 = TCP Open Connection(address="192.168.101.108", remote port or service name=u16 3502) -> (connection ID=w126:refnum<k5>, error out=w121:errorcluster)  [unwired: 3 in]
        n217 = case shown="No Error" w121 {
          selector: w121 -> [w131 w158]
          tunnel: w126 -> [w136 w159]
          tunnel: [w135 w159] -> w125
          tunnel: [w134 w158] -> w124
          tunnel: [w133 w157] -> w123
          tunnel: w120 -> [w130 _]
          tunnel: w119 -> [w129 _]
          frame No Error {
            n218 = node-c288() -> (w138:T3)  [unwired: 4 in]
            n219 = timed-loop {
              tunnel: w136 -> [w152]
              tunnel: w131 -> [w151]
              tunnel: [w150] -> w135
              tunnel: [w149] -> w134
              tunnel: [w141] -> w133
              shift-right: [w143] -> _
              shift-left: FALSE -> [w146]
              timing: w138 -> [_]
              timing-out: [_] -> w137
              tunnel: w130 -> [w140]
              tunnel: w129 -> [w139]
              stop <- w147 stop-if-true
              n220 = node-c288() -> ()  [unwired: 1 in, 1 out]
              n221 = Dequeue Element(queue=w140, error in (no error)=w139) -> (element=w142:string)  [unwired: 1 in, 3 out]
              n222 = Select(t=FALSE, s=w146, f=TRUE) -> (s? t:f=w143:bool)
              "TCP packet\nSend To SEPTIC" <- w143
              n223 = TCP Write(connection ID=w152, data in=w142, error in (no error)=w151) -> (connection ID out=w150:refnum<k5>, error out=w149:errorcluster)  [unwired: 1 in, 1 out]
              n224 = local read "stop"() -> (w141:bool)
              n225 = Unbundle(w149) -> ("status"=w148:bool)  [unwired: 2 out]
              n226 = node-c288() -> ()  [unwired: 1 in, 1 out]
              n227 = Compound Arithmetic op=OR(w148, w141) -> (w147:bool)
            }
            n228 = node-c288(w137) -> ()  [unwired: 1 out]
          }
          frame Error {
            n229 = local read "stop"() -> (w157:bool)
          }
        }
        n230 = TCP Close Connection(connection ID=w125, error in (no error)=w124) -> (error out=→"SEPTIC TCP Error Out":errorcluster)  [unwired: 1 in, 1 out]
        n231 = Wait (ms)(milliseconds to wait=u32 1000) -> ()  [unwired: 1 out]
      }
      n232 = node-c288(w50) -> ()  [unwired: 1 out]
    }
    frame Error {
    }
  }
  n233 = VISA Close(VISA resource name=w25, error in (no error)=w26) -> (error out=→"Serial error out":errorcluster)
